vi "Get Channel Data in By Channel ID (offline).vi"(8 "error in (no error)":errorcluster, 9 "Channel IDs":T1[](array[typedef]) format="%.0x", 11 "Device Ref in":T1 format="%.0x") -> (0 "error out":errorcluster, 1 "Default Values":dbl[](array[numeric]), 2 "FIFO Indices":i32[](array[numeric]), 3 "Device Ref out":T1 format="%.0x", 4 "Channel Names":string[](array[string]))   [LabVIEW 2020, in "Routing and Faulting System Explorer.lvlib"]
uses:
  Routing and Faulting System Explorer.lvlib
  <vilib>/NI VeriStand/Custom Device API/Custom Device Item Ref.ctl
  <vilib>/NI VeriStand/Custom Device API/Custom Device API.lvlib
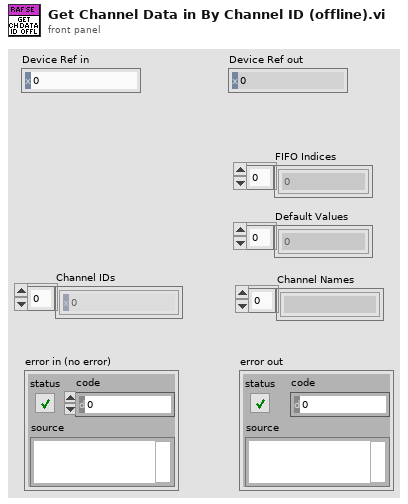
[diagram p1: front panel]
types:
  T1 = typedef "Custom Device API.lvlib/Custom Device Item Ref.ctl" = u64
  T2 = typedef "Custom Device API.lvlib/Custom Device Channel.ctl" = cluster{"Type":T3, "Units":string, "Default Value":dbl, "Faultable":bool, "Scalable":bool}
  T3 = typedef "Custom Device API.lvlib/Custom Device Channel Type.ctl" = enum16{"Input", "Output"}
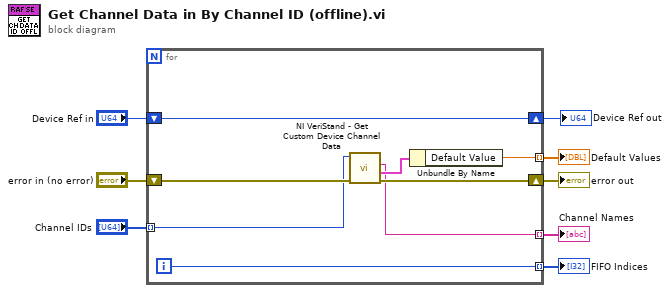
[diagram p0: block diagram]
diagram:
  n1 = for {
    shift-right: [w16] -> w7
    shift-left: "error in (no error)" -> [w12]
    tunnel: "Channel IDs" -> [w10] mode=indexing
    tunnel: [w14] -> w8 mode=indexing
    tunnel: [w13] -> w5 mode=indexing
    tunnel: [w9] -> w4 mode=indexing
    shift-right: [w11] -> w1
    shift-left: "Device Ref in" -> [w11]
    i -> [w9]
    n2 = call <vilib>:"NI VeriStand - Get Custom Device Channel Data.vi"("error in (no error)"=w12, "Channel Ref in"=w10) -> ("error out"=w16:errorcluster, "Channel"=w15:T2, "Channel Name"=w13:string)  [unwired: 4 in, 3 out]
    n3 = Unbundle By Name(w15) -> ("Default Value"=w14:dbl)
  }
  "Default Values" <- w8
  "error out" <- w7
  "FIFO Indices" <- w4
  "Channel Names" <- w5
  "Device Ref out" <- w1
